vi "Init.vi"(8 "error in (no error)":errorcluster, 10 "Error Log Path":path, 11 "Text Log in":refnum<class "XML Log.lvclass">) -> (0 "error out":errorcluster, 3 "Text Log out":refnum<class "XML Log.lvclass">)   [LabVIEW 2020, in "Error Log Classes.lvlib" / "XML Log.lvclass"]
uses:
  XML Log.lvclass
  XML Log.lvclass/XML Log.ctl
  <vilib>/xml/Close Reference(Node).vi
  <vilib>/xml/NI_XML.lvlib
  Error Log/Error Log.lvclass
  <resource>/objmgr/DOMUserDefRef.rc
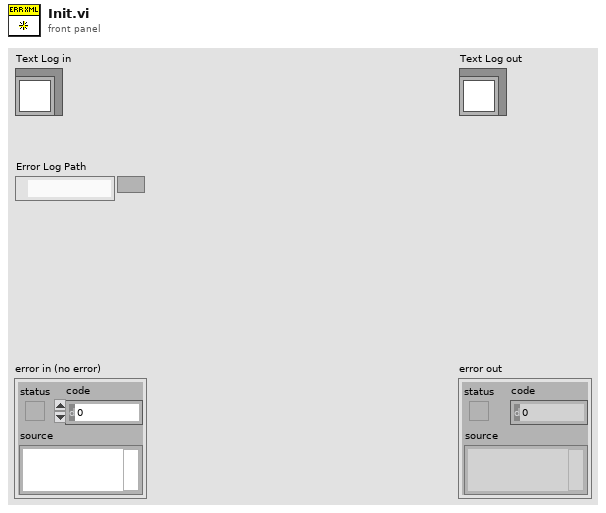
[diagram p1: front panel]
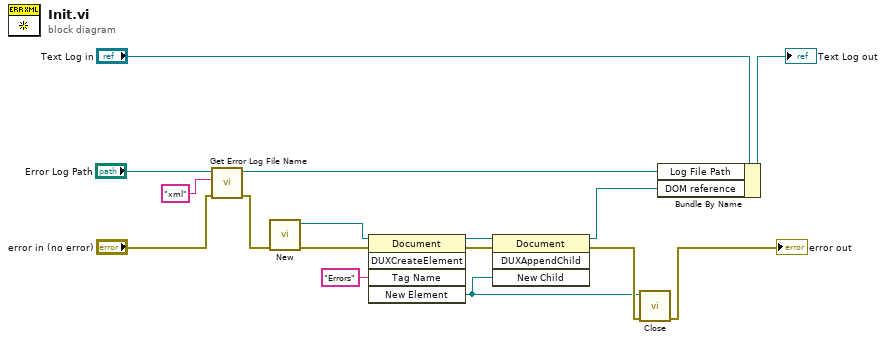
[diagram p0: block diagram]
diagram:
  n1 = call "Get Error Log File Name.vi"("error in (no error)"="error in (no error)", "Extension"="xml", "Error Log Path in"="Error Log Path") -> ("error out"=w11:errorcluster, "Error Log Path out"=w13:path)  [unwired: 7 in]
  n2 = call <vilib>:"New.vi"("error in (no error)"=w11) -> ("error out"=w7:errorcluster, "DOM document out"=w6:refnum<k20>)  [unwired: 7 in]
  n3 = invoke class="Document" method="DUXCreateElement"(reference=w6, error in=w7, "Tag Name"="Errors") -> (reference out=w9:refnum<k20>, error out=w8:errorcluster, "New Element"=w1:refnum<k20>)  [unwired: 2 in, 2 out]
  n4 = invoke class="Document" method="DUXAppendChild"(reference=w9, error in=w8, "New Child"=w1) -> (reference out=w5:refnum<k20>, error out=w3:errorcluster)  [unwired: 1 in, 2 out]
  n5 = call-poly <vilib>:"Close.vi"("error in (no error)"=w3, "node"=w1) -> ("error out"=→"error out":errorcluster)  [unwired: 7 in]
  n6 = Bundle By Name(cluster="Text Log in", "Log File Path"=w13, "DOM reference"=w5) -> (→"Text Log out":refnum<class "XML Log.lvclass">)
